vi "CheckTime.vi"(7 "target time":dbl, 9 "start index":i32, 10 "acquiredSeconds":dbl, 11 "DVR element in":T1) -> (1 "stop index (include)":i32, 2 "time met":bool, 4 "seconds of data":dbl)   [LabVIEW 2017, in "DataAccumulator.lvlib"]
uses:
  <vilib>/addons/InsightCM/Devices/Shared/Common/DataAccumulator/DataAccumulator.lvlib
  <vilib>/addons/InsightCM/Devices/Shared/Common/DVRBuffer/controls/DVRElement.ctl
  <vilib>/addons/InsightCM/Devices/Shared/Common/DVRBuffer/DVRBuffer.lvlib
panel:
  # "if zero, use entire block"
  # "Seconds of data from start index to stop index.\nif not enough data (stop index = 0), this is the\nseconds of data from start index through the \nend of the block."
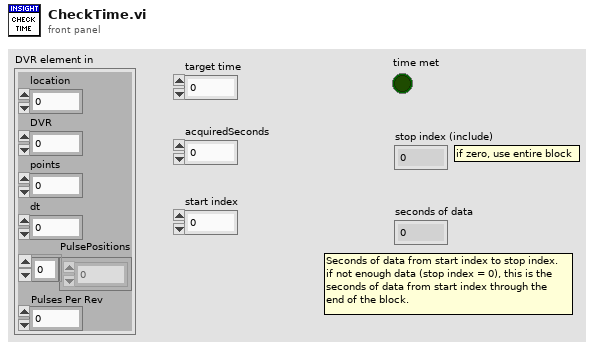
[diagram p1: front panel]
types:
  T1 = typedef "DVRBuffer.lvlib/DVRElement.ctl" = cluster{"location":u32, "DVR":u32, "points":i32, "dt":dbl, "PulsePositions":dbl[], "Pulses Per Rev":dbl}
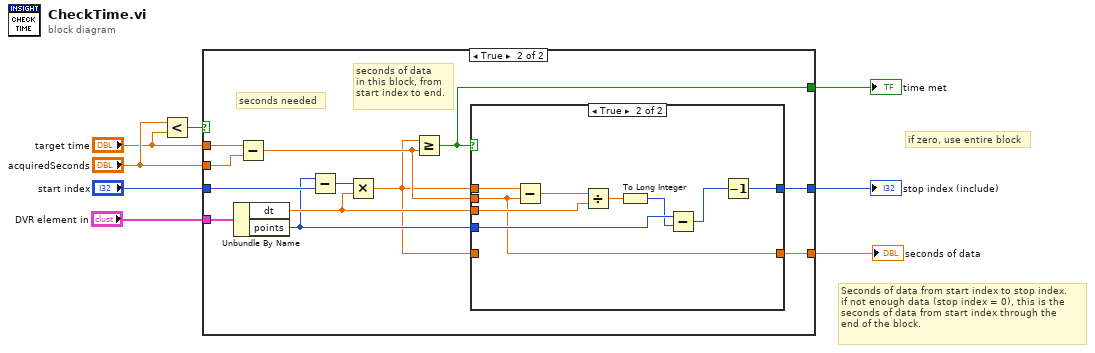
[diagram p0: block diagram]
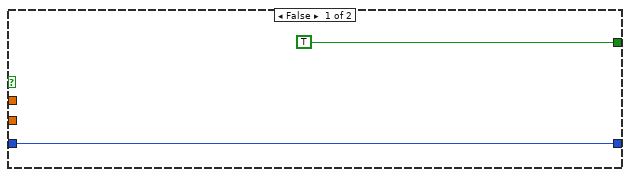
[diagram p2: hidden frame]
diagram:
  # "Seconds of data from start index to stop index.\nif not enough data (stop index = 0), this is the\nseconds of data from start index through the \nend of the block."
  # "if zero, use entire block"
  n1 = Less?(x="acquiredSeconds", y="target time") -> (x < y?=w2:bool)
  n2 = case shown="True" w2 {
    tunnel: "start index" -> [w9 w20]
    tunnel: [TRUE w19] -> w7
    tunnel: "DVR element in" -> [_ w16]
    tunnel: [w9 w15] -> w5
    tunnel: "acquiredSeconds" -> [_ w14]
    tunnel: "target time" -> [_ w13]
    tunnel: [_ w12] -> w1
    frame False {
    }
    frame True {
      # "seconds of data\nin this block, from\nstart index to end."
      # "seconds needed"
      n3 = Unbundle By Name(w16) -> ("dt"=w22:dbl, "points"=w17:i32)
      n4 = Subtract(x=w13, y=w14) -> (x-y=w18:dbl)
      n5 = Subtract(x=w17, y=w20) -> (x-y=w21:i32)
      n6 = Multiply(x=w21, y=w22) -> (x*y=w11:dbl)
      n7 = Greater Or Equal?(x=w11, y=w18) -> (x >= y?=w19:bool)
      n8 = case shown="True" w19 {
        tunnel: w11 -> [_ w25]
        tunnel: w22 -> [_ w32]
        tunnel: w18 -> [_ w24]
        tunnel: w17 -> [_ w30]
        tunnel: [_ w27] -> w15
        tunnel: [w23 w24] -> w12
        tunnel: w11 -> [w23 _]
        frame False {
          # "not enough points"
          # "Not enough points"
        }
        frame True {
          # "Too many points"
          n9 = Subtract(x=w25, y=w24) -> (x-y=w26:dbl)
          n10 = Divide(x=w26, y=w32) -> (x/y=w31:dbl)
          n11 = To Long Integer(number=w31) -> (32bit integer=w29:i32)
          n12 = Subtract(x=w30, y=w29) -> (x-y=w28:i32)
          n13 = Decrement(x=w28) -> (x-1=w27:i32)
        }
      }
    }
  }
  "time met" <- w7
  "stop index (include)" <- w5
  "seconds of data" <- w1
